vi "Pachube Update Feed LaunchPad.vi"(5 "Pachube datastream ID":string="0", 6 "Format":string(combo), 7 "timeout ms (60000)":i32=60000, 8 "error in (no error)":errorcluster, 9 "Pachube API Key":string, 10 "Pachube feed ID":string, 11 "Data":string) -> (0 "error out":errorcluster, 1 "Error code":i32, 2 "Error":bool)   [LabVIEW 2010]
doc: "Example of using standard HTTP PUT method with LabVIEW TCP/IP vi's to send data to Pachube.\n\nPachube is a service that enables you to connect, tag and share real time sensor data from objects, devices, buildings and environments around the world. The key aim is to facilitate interaction between remote environments, both physical and virtual. Check out the details of the service at www.pachube.com\n\nThis vi is was created by modifying Bjornar Svingen's Twitter Update Status vi (bjornar.svingen@sintef.no bjornar.svingen@ktv.no).\n\nTo access the Pachube service (which is still beta) you will need an invitation and an API Key - which you can request on the site.\n\nOnce you are logged in - you need to create an empty manual feed. This will get you the URL's for your feed in the form www.pachube.com/api/1234.csv for CSV or www.pachube.com/api/1234.xml for EEML. The simplest data format is CSV(ie just a list of values like 10.1,20.3,30.2). In this case after the first update using this format you can edit your feed on the site to name each item. EEML is an XML formatted data format which allows you to include meta data such as item names. See www.eeml.org for examples. A simple exmple is shown below:\n \n<?xml version=\"1.0\" encoding=\"UTF-8\"?>\n<eeml xmlns=\"http://www.eeml.org/xsd/005\">\n <environment>\n <data id=\"0\">\n <tag>Power</tag>\n <value>1000</value>\n <unit symbol=\"W\" type=\"derivedSI\">watt</unit>\n </data>\n <data id=\"1\">\n <tag>Temperature</tag>\n <value>21.5</value>\n <unit symbol=\"C\" type=\"derivedSI\">degrees Celsius</unit>\n </data>\n </environment>\n</eeml>\n\nEEML will automaticlly configure your feed with item names.\n\nIan Bell\nian.bell@ni.com"
panel:
  out "resulting string":string
  out "HTML source":string caption="HTTP response"
  # "(in EEML for EEML feed or JSON for JSON feed)"
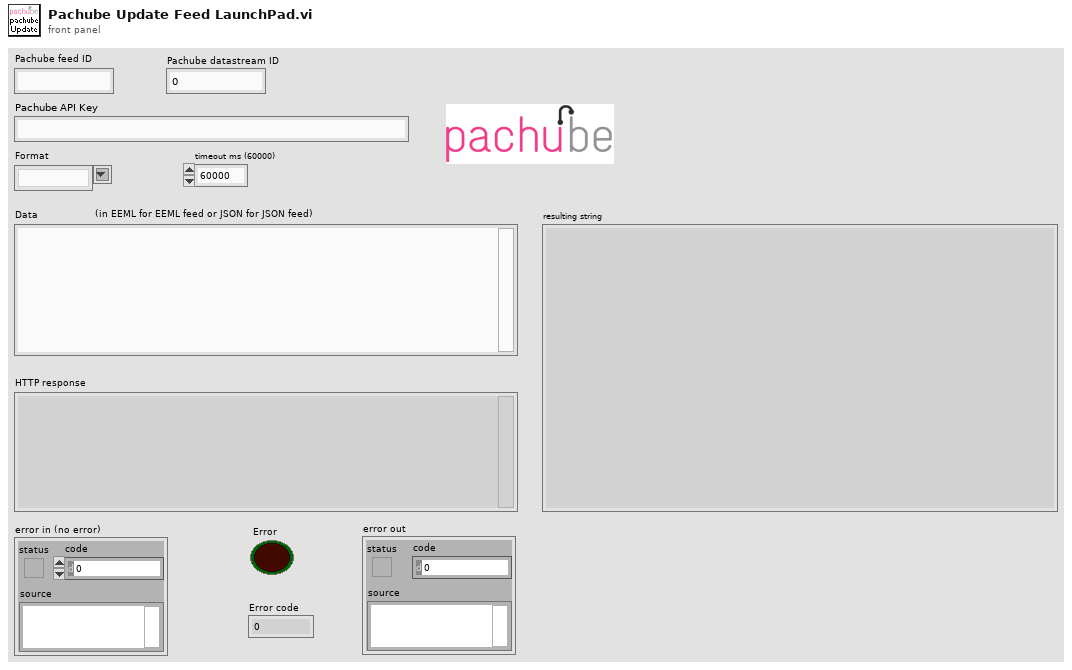
[diagram p1: front panel]
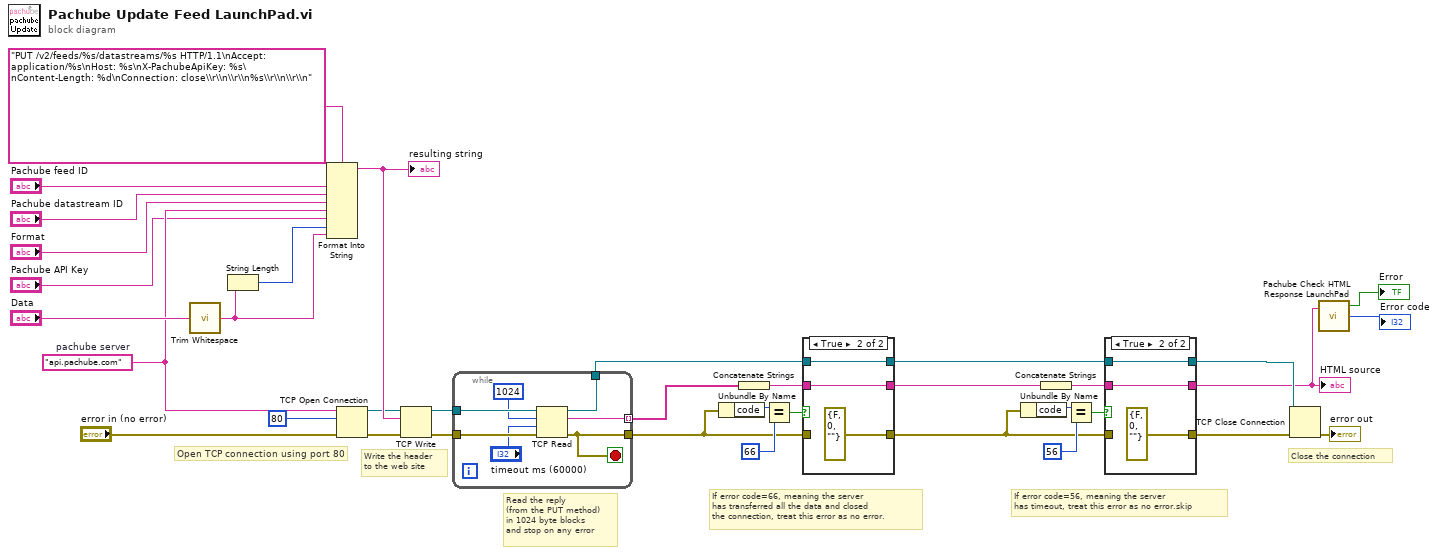
[diagram p0: block diagram]
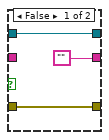
[diagram p2: hidden frame]
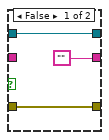
[diagram p3: hidden frame]
diagram:
  w13 = "api.pachube.com"  # pachube server
  # "If error code=56, meaning the server\nhas timeout, treat this error as no error.skip"
  # "Close the connection"
  # "If error code=66, meaning the server\nhas transferred all the data and closed\nthe connection, treat this error as no error."
  # "Read the reply\n(from the PUT method)\nin 1024 byte blocks\nand stop on any error"
  # "Write the header\nto the web site"
  # "Open TCP connection using port 80"
  n1 = call <vilib>:"Trim Whitespace.vi"("string"="Data") -> ("trimmed string"=w16:string)  [unwired: 1 in]
  n2 = String Length(string=w16) -> (length=w17:i32)
  n3 = Format Into String(format string="PUT /v2/feeds/%s/datastreams/%s HTTP/1.1\nAccept: application/%s\nHost: %s\nX-PachubeApiKey: %s\nContent-Length: %d\nConnection: close\\r\\n\\r\\n%s\\r\\n\\r\\n" ("Command"), "Pachube feed ID", "Pachube datastream ID", "Format", w13, "Pachube API Key", w17, w16) -> (resulting string=w36:string)  [unwired: 2 in, 1 out]
  "resulting string" <- w36
  n4 = TCP Open Connection(address=w13, remote port or service name=u16 80 ("remote port"), error in (no error)="error in (no error)") -> (connection ID=w31:refnum<k5>, error out=w32:errorcluster)  [unwired: 2 out]
  n5 = TCP Write(connection ID=w31, data in=w36, error in (no error)=w32) -> (connection ID out=w28:refnum<k5>, error out=w27:errorcluster)  [unwired: 2 out]
  n6 = while {
    tunnel: w27 -> [w43]
    tunnel: w28 -> [w42]
    tunnel: [w38] -> w25
    tunnel: [w41] -> w22
    tunnel: [w40] -> w24 mode=indexing
    stop <- w38 stop-if-true
    n7 = TCP Read(connection ID=w42, bytes to read=1024, error in (no error)=w43, 9:"timeout ms (60000)") -> (connection ID out=w41:refnum<k5>, data out=w40:string, error out=w38:errorcluster)  [unwired: 1 out]
  }
  n8 = Unbundle By Name(w25) -> ("code"=w30:i32)
  n9 = Concatenate Strings(w24) -> (w23:string)
  n10 = Equal?(x=w30, y=66) -> (x = y?=w29:bool)
  n11 = case shown="True" w29 {
    tunnel: ["" w48] -> w5
    tunnel: w23 -> [_ w48]
    tunnel: [w45 errorcluster {"status"=FALSE, "code"=0, "source"=""} ("error in (no error)")] -> w4
    tunnel: w25 -> [w45 _]
    tunnel: w22 -> [w44 w47]
    tunnel: [w44 w47] -> w6
    frame False {
    }
    frame True {
    }
  }
  n12 = Unbundle By Name(w4) -> ("code"=w10:i32)
  n13 = Concatenate Strings(w5) -> (w7:string)
  n14 = Equal?(x=w10, y=56) -> (x = y?=w9:bool)
  n15 = case shown="True" w9 {
    tunnel: ["" w54] -> w2
    tunnel: w7 -> [_ w54]
    tunnel: [w51 errorcluster {"status"=FALSE, "code"=0, "source"=""} ("error in (no error)")] -> w1
    tunnel: w4 -> [w51 _]
    tunnel: w6 -> [w50 w53]
    tunnel: [w50 w53] -> w3
    frame False {
    }
    frame True {
    }
  }
  "HTML source" <- w2
  n16 = TCP Close Connection(connection ID=w3, error in (no error)=w1) -> (error out=→"error out":errorcluster)  [unwired: 2 out]
  n17 = call "Pachube Check HTML Response LaunchPad.vi"("HTML Response"=w2) -> ("Error"=→"Error":bool, "Error code"=→"Error code":i32)  [unwired: 1 in, 1 out]
